vi "Read Role.vi"(8 "error in (no error)":errorcluster, 11 "Personnel in":refnum<class "Personnel.lvclass">) -> (0 "error out":errorcluster, 2 "Type":T1, 3 "Personnel out":refnum<class "Personnel.lvclass">)   [LabVIEW 2015, in "Personnel.lvclass"]
uses:
  Personnel.lvclass
  PersonnelType.ctl
  Personnel.lvclass/Personnel.ctl
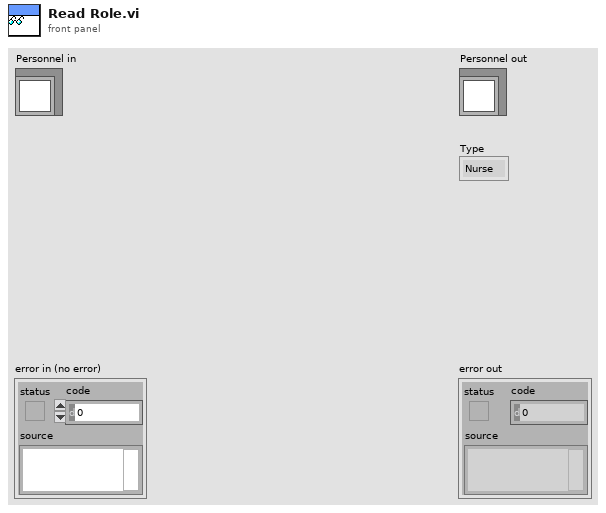
[diagram p1: front panel]
types:
  T1 = typedef "Personnel.lvclass/PersonnelType.ctl" = enum16{"Nurse", "Doctor", "Cleanning", "Admin"}
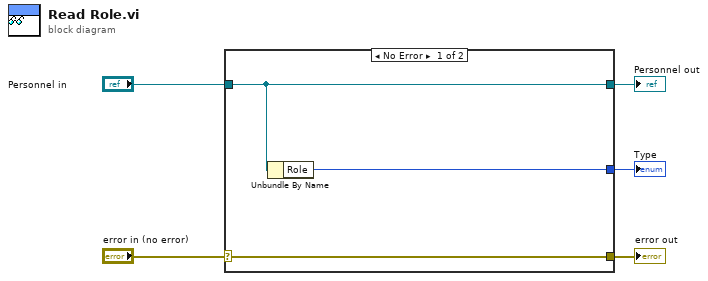
[diagram p0: block diagram]
diagram:
  n1 = case shown="No Error" "error in (no error)" {
    selector: "error in (no error)" -> [w8 w9]
    tunnel: [w8 w9] -> w4
    tunnel: [w7 w10] -> w2
    tunnel: "Personnel in" -> [w7 w10]
    tunnel: [w6 _] -> w1
    frame No Error {
      n2 = Unbundle By Name(w7) -> ("Role"=w6:T1)
    }
    frame Error {
    }
  }
  "error out" <- w4
  "Personnel out" <- w2
  "Type" <- w1
